vi "UpdatedEnumControls_new.vi"(7 "Seasons":T3(ring)=enum."Rainy", 10 "Months":T1(ring)=enum."October", 11 "Colors":T2(ring)=enum."Red") -> ()   [LabVIEW 2015]
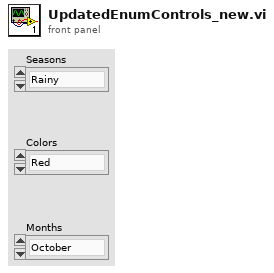
[diagram p1: front panel]
types:
  T1 = enum32{"NorFeb", "LeapFeb", "January", "February", "March", "April", "May", "June", "July", "August", "September", "October", "November", "December"}
  T2 = enum16{"Crimson", "Red", "Green", "Blue", "Yellow", "pervench", "Purple", "Orange"}
  T3 = enum32{"Foggy", "Rainy", "Fall", "Winter", "Spring", "Summer"}
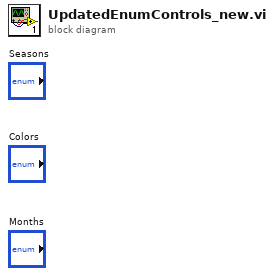
[diagram p0: block diagram]
diagram:
